vi "find_PrepLineObj_InstObj_by_name.vi"(8 "error in (no error)":errorcluster, 11 "PrepLineObject Name":string) -> (0 "error out":errorcluster, 1 "found?":bool, 2 "found InstrObject out":refnum<class "instrument.lvclass">, 3 "found PrepLineObject out":refnum<class "PrepLineObject.lvclass">)   [LabVIEW 2017]
doc: "finds the PrepLineObject and Instrument taht belongs to this object by the name of the PrepLineObject"
uses:
  Classes/PrepLineObject/PrepLineObject.lvclass
  Classes/Instrument/instrument.lvclass
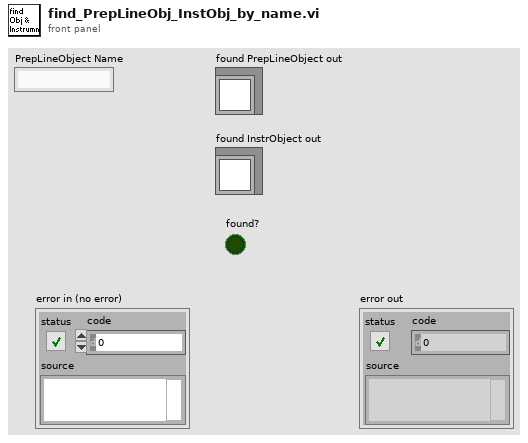
[diagram p1: front panel]
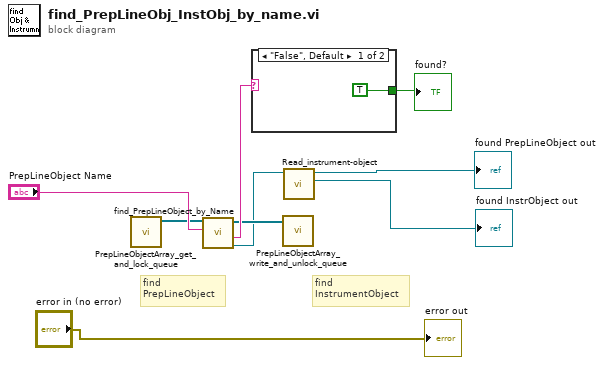
[diagram p0: block diagram]
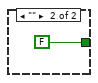
[diagram p2: hidden frame]
diagram:
  # "find\nInstrumentObject"
  # "find\nPrepLineObject"
  n1 = call "PrepLineObjectArray_get_and_lock_queue.vi"() -> ("PrepLineObjects"=w3:refnum<class "PrepLineObject.lvclass">[])  [unwired: 10 in, 1 out]
  n2 = call "find_PrepLineObject_by_Name.vi"("Name of Object"="PrepLineObject Name", "PrepLineObjects in"=w3) -> ("found PrepLineObject"=w1:refnum<class "PrepLineObject.lvclass">, "instrument"=w8:string, "PrepLineObjectsOut"=w2:refnum<class "PrepLineObject.lvclass">[])  [unwired: 3 in, 3 out]
  n3 = case shown="\"False\", Default" w8 {
    tunnel: [TRUE FALSE] -> w7
    frame "False", Default {
    }
    frame "" {
    }
  }
  "found?" <- w7
  n4 = call "PrepLineObjectArray_write_and_unlock_queue.vi"("PrepLineObjArray"=w2) -> ()  [unwired: 10 in, 1 out]
  n5 = call-dynamic "Read_instrument-object.vi"("PrepLineObject in"=w1) -> ("instrument.lvclass"=→"found InstrObject out":refnum<class "instrument.lvclass">, "PrepLineObject out"=→"found PrepLineObject out":refnum<class "PrepLineObject.lvclass">)  [unwired: 8 in, 1 out]
  "error out" <- "error in (no error)"
